vi "Storage Factory.vi"(8 "error in (no error)":errorcluster, 11 "VolatusConfig in":refnum<class "VolatusConfig.lvclass">) -> (0 "error out":errorcluster, 2 "Storage":refnum<class "Config Storage.lvclass">, 3 "VolatusConfig out":refnum<class "VolatusConfig.lvclass">)   [LabVIEW 2020, in "VolatusConfig.lvlib" / "VolatusConfig.lvclass"]
uses:
  VolatusConfig.lvclass
  VolatusConfig.lvclass/VolatusConfig.ctl
  VolatusConfig.lvlib
  lv-cdm/CDM-Config/Config Storage/Config Storage.lvclass
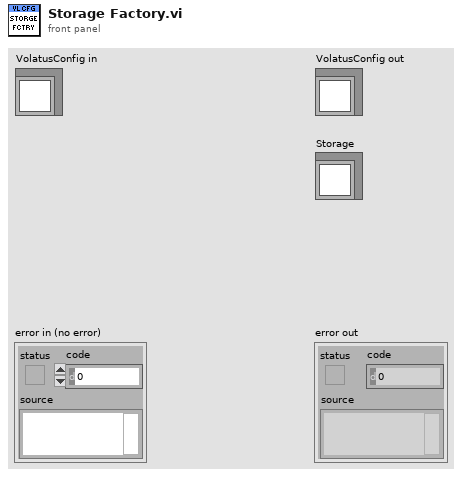
[diagram p1: front panel]
types:
  T1 = typedef "VolatusConfig.lvlib/Config Format.ctl" = enum16{"JSON", "INI", "SQLite"}
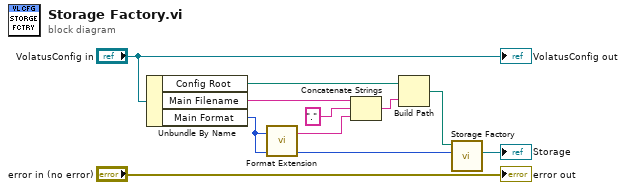
[diagram p0: block diagram]
diagram:
  n1 = Unbundle By Name("VolatusConfig in") -> ("Config Root"=w6:path, "Main Filename"=w8:string, "Main Format"=w2:T1)
  n2 = call "Format Extension.vi"("Format"=w2) -> ("Extension"=w4:string)  [unwired: 2 in]
  n3 = Concatenate Strings(w8, "." ("string"), w4) -> (w5:string)
  n4 = Build Path(base path=w6, name or relative path=w5) -> (appended path=w3:path)
  n5 = call "Storage Factory.vi"("Format"=w2, "Config Path"=w3) -> ("Storage"=→"Storage":refnum<class "Config Storage.lvclass">)  [unwired: 9 in]
  "error out" <- "error in (no error)"
  "VolatusConfig out" <- "VolatusConfig in"
